vi "Destroy Spy.vi"(8 "error in (no error)":errorcluster, 11 "LabSpy":refnum<data-value>) -> (0 "error out":errorcluster)   [LabVIEW 2013, in "LabSpy.lvclass"]
doc: "Delete the spy object and release any resources."
uses:
  LabSpy.lvclass
  LabSpy.lvclass/LabSpy.ctl
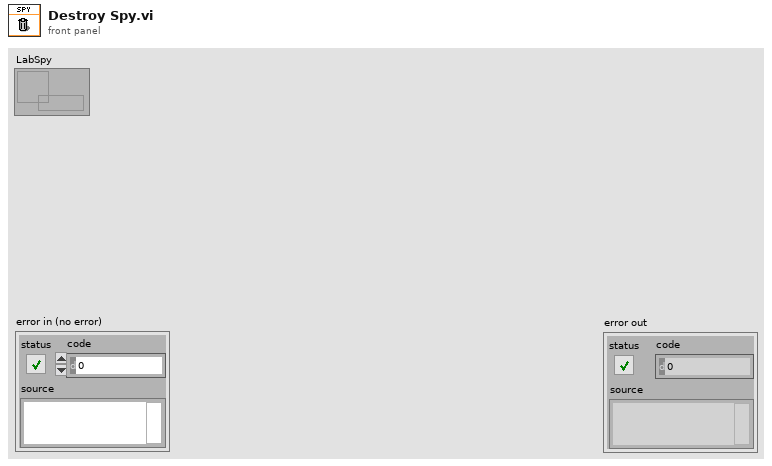
[diagram p1: front panel]
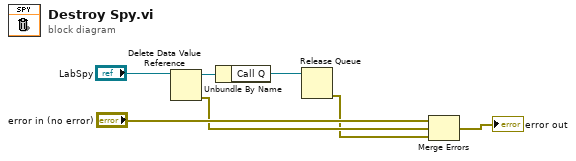
[diagram p0: block diagram]
diagram:
  n1 = Delete Data Value Reference(data value reference="LabSpy") -> (data value=w3:refnum<class "LabSpy.lvclass">, error out=w5:errorcluster)  [unwired: 1 in]
  n2 = Unbundle By Name(w3) -> ("Call Q"=w2:refnum<queue>)
  n3 = Release Queue(queue=w2) -> (error out=w1:errorcluster)  [unwired: 2 in, 2 out]
  n4 = Merge Errors("error in (no error)", w5, w1) -> (→"error out":errorcluster)
